vi "sub_cyclic_prefixer.vi"(8 "FFT size":i32=256, 9 "CP length":i32=64, 11 "time_samples":cdb[](array[numeric])) -> (3 "cp ofdm symbol":cdb[](array[numeric]))   [LabVIEW 2014]
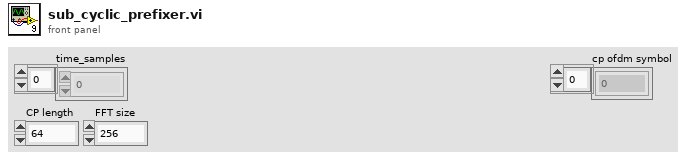
[diagram p1: front panel]
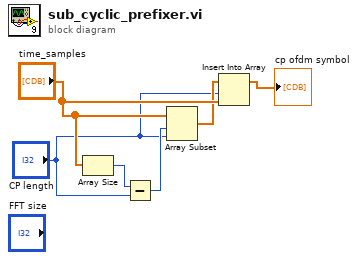
[diagram p0: block diagram]
diagram:
  n1 = Array Size(array="time_samples") -> (size(s)=w5:i32)
  n2 = Subtract(x=w5, y="CP length") -> (x-y=w6:i32)
  n3 = Array Subset(array="time_samples", index=w6, length="CP length") -> (w2:cdb[])
  n4 = Insert Into Array(array=w2, index="CP length", new element="time_samples") -> (→"cp ofdm symbol":cdb[])
